vi "LakeShore 340 Controller.vi"(0 "GBPIB Address":refnum<visa-resource-name>, 1 "Reset (I) (0.0)":dbl min=0.0 max=1000.0 step=0.1 format="%.1f", 2 "Rate (D) (0)":dbl min=0.0 max=1000.0 step=1.0, 3 "Manual Output (0.00)":dbl min=0.0 max=100.0 step=0.01 format="%.2f", 4 "Heater Range (0: Off)":u16(ring) items=["Off", "1", "2", "3", "4", "5"], 5 "error out":errorcluster, 6 "Gain (P) (0.0)":dbl min=0.0 max=1000.0 step=0.1 format="%.1f", 7 "Setpoint (0.0)":dbl min=-273.0 max=300000.0 step=0.0001 format="%#.2g", 8 "Loop (0: 1)":u16(ring) items=["1", "2"], 9 "Input (0: A)":u16(ring) items=["A", "B", "C", "D"], 10 "Delay After Config":u32=1000 min=1000 max=99999 step=1) -> (14 "GBPIB Address 2":refnum<visa-resource-name>, 15 "Celsius":dbl min=-273.16 max=1372.0 step=1e-05 format="%#_5g", 16 "K":dbl min=0.0 max=1645.0 step=1e-05 format="%^#_5g", 17 "Ohm":dbl min=-7.5 max=300000.0 step=1e-05 format="%^#_6g", 18 "Heater Output":dbl(slide) min=0.0 max=100.0 step=0.01 scale=0.0..100.0 scale format="%.2f", 19 "error":errorcluster)   [LabVIEW 2019]
doc: "This VI was designed to demonstrate typical usage of sub vi's containing the more common 340 functions.\n\nThis example configures the loop and setpoint of the instrument, allows for a delay, and then reads sensor and heater output data. The user is given the option of just reading data and not configuring the instrument."
uses:
  NHMFL Optics/Globals and TypeDefs/Type Definitions.llb/3 way Status.ctl
  <vilib>/Analysis/baseanly.llb/Mean (DBL).vi
  <vilib>/Analysis/2dsp.llb/Power Spectrum (DBL).vi
  NHMFL Optics/Globals and TypeDefs/gStatus.vi
  NHMFL Optics/Globals and TypeDefs/gTemperature.vi
  <vilib>/Analysis/NI_AALPro.lvlib
  <vilib>/Analysis/NI_AALBase.lvlib
panel:
  out "K plot_t":dbl(graph)
  out "K plot":dbl(graph)
  in  "Tab Control":enum32{"Temperatures", "Configuration", "Misc"}(tab)
  in  "Tolerance":dbl=0.1 min=-273.0 max=300000.0 step=0.0001 format="%#.2g"
  out "Temperature":T1(graph)
  in  "Pause Reading":bool
  in  "AbortChangeTemp":bool
  in  "Reading Rate (ms)":u32=500
  in  "CalibrationTable":bool
  in  "Time-out (s)":dbl
  in  "Manual Advancing":bool
  in  "SetPID":bool
  out "Temperature Control state":T2(ring)
  out "XY Graph":cluster{dbl[], dbl[]}(graph)
  out "Peak time (point)":dbl
  in  "FFT":bool
  in  "stop":bool
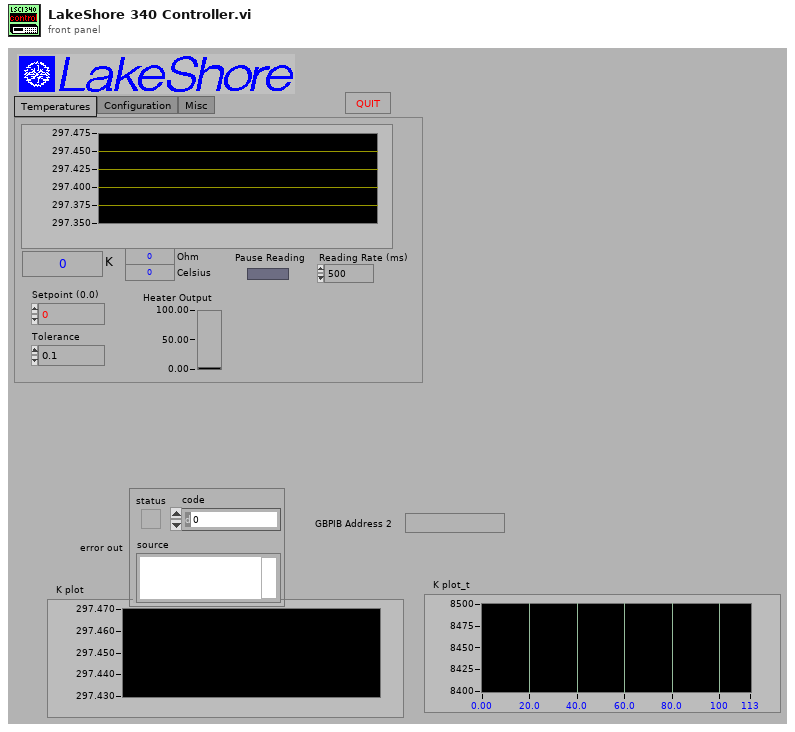
[diagram p1: front panel]
types:
  T1 = cluster{"History Data":dbl[], "History Data":dbl[]}
  T2 = enum16{"--Quit--", "Error", "Init", "Ready", "Set PID", "Set Setpoint", "Curve Manager"}
  T3 = typedef "3 way Status.ctl" = u8
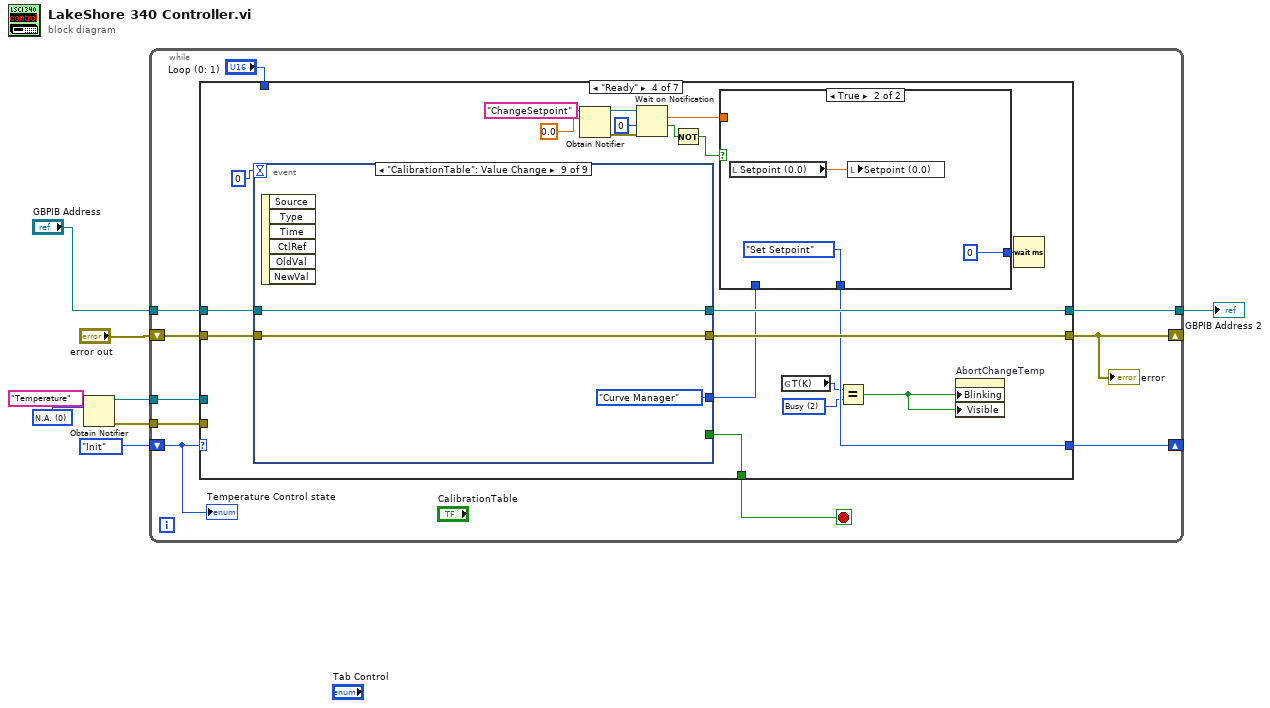
[diagram p0: block diagram]
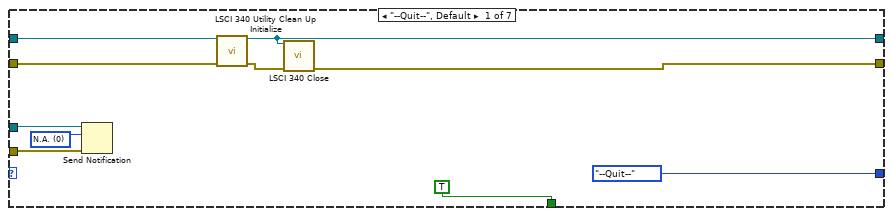
[diagram p2: hidden frame]
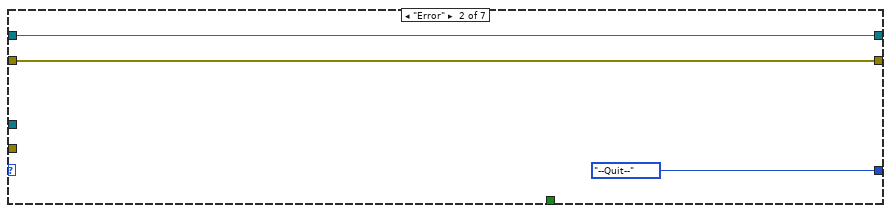
[diagram p3: hidden frame]
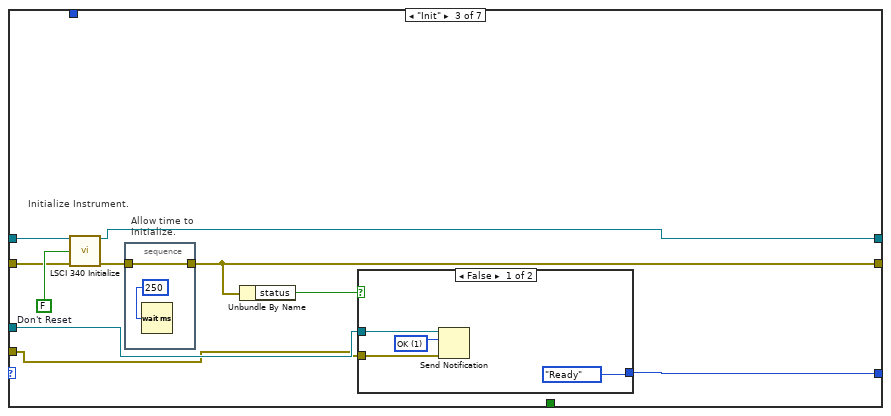
[diagram p4: hidden frame]
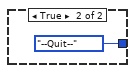
[diagram p5: hidden frame]
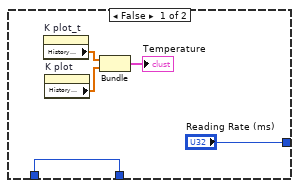
[diagram p6: hidden frame]
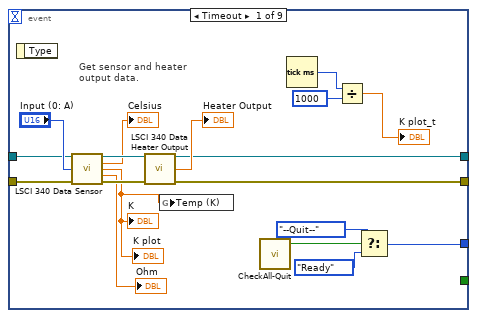
[diagram p7: hidden frame]
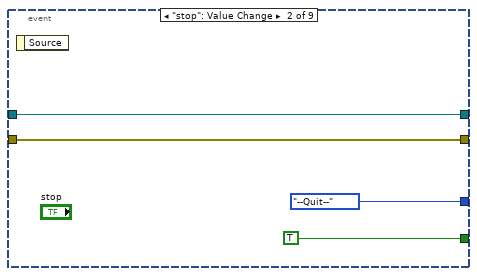
[diagram p8: hidden frame]
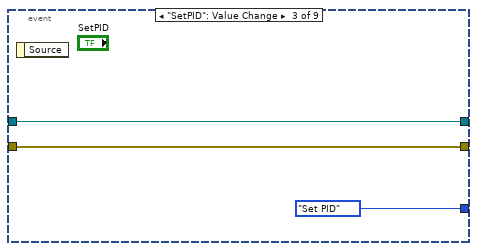
[diagram p9: hidden frame]
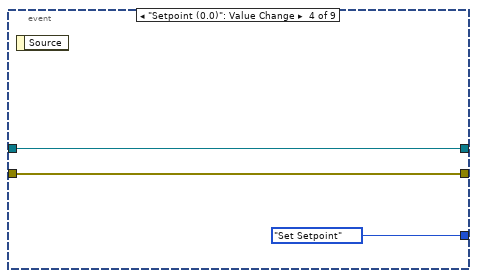
[diagram p10: hidden frame]
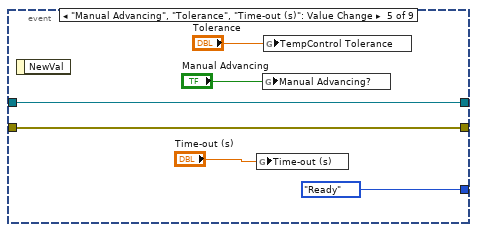
[diagram p11: hidden frame]
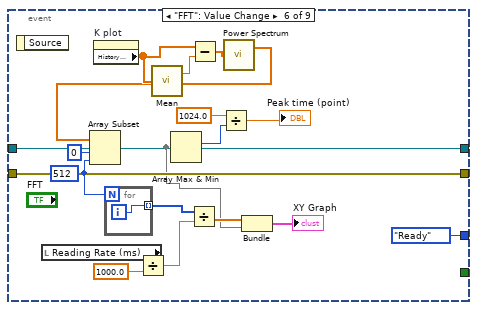
[diagram p12: hidden frame]
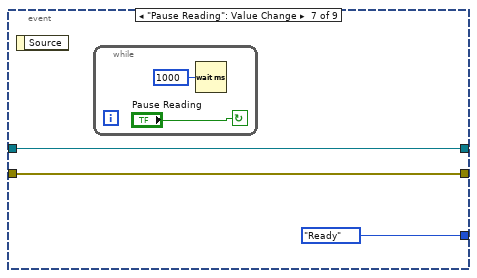
[diagram p13: hidden frame]
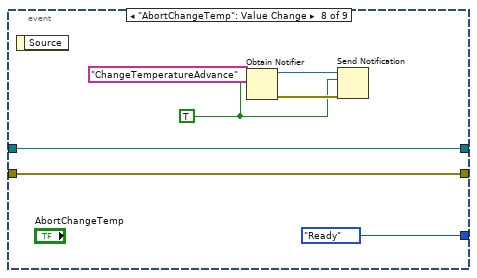
[diagram p14: hidden frame]
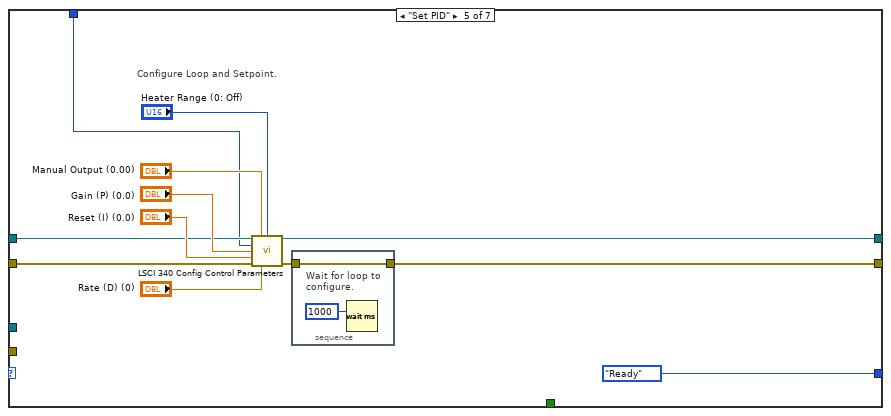
[diagram p15: hidden frame]
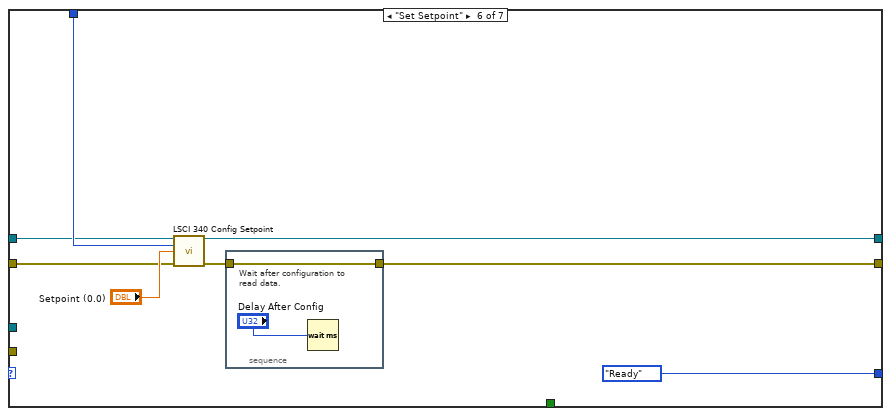
[diagram p16: hidden frame]
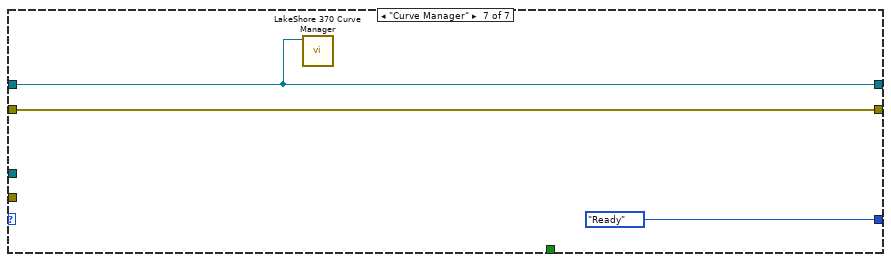
[diagram p17: hidden frame]
diagram:
  w7 = T3 0 items=["N.A.", "OK", "Busy", "Done"] ("Saving")
  n1 = Obtain Notifier(name (unnamed)="Temperature", notification data type=w7) -> (notifier out=w5:refnum<notifier>, error out=w4:errorcluster)  [unwired: 2 in, 1 out]
  n2 = while {
    tunnel: "GBPIB Address" -> [w18]
    shift-right: [w15] -> _
    shift-left: "error out" -> [w17]
    tunnel: [w14] -> w1
    shift-right: [w13] -> _
    shift-left: T2."Init" ("Temperature Control state") -> [w12]
    tunnel: w5 -> [w10]
    tunnel: w4 -> [w9]
    stop <- w11 stop-if-true
    n3 = case shown="\"Ready\"" w12 {
      tunnel: w17 -> [w24 w30 w39 w68 w157 w165 w172]
      tunnel: w18 -> [w25 w31 w33 w67 w153 w163 w170]
      tunnel: [w28 w30 w38 w65 w148 w161 w172] -> w15
      tunnel: [w23 w31 w32 w66 w147 w162 w170] -> w14
      tunnel: "Loop (0: 1)" -> [_ _ _ _ w149 w164 _]
      tunnel: [T2."--Quit--" ("Temperature Control state") T2."--Quit--" ("Temperature Control state") w36 w53 T2."Ready" ("Temperature Control state") T2."Ready" ("Temperature Control state") T2."Ready" ("Temperature Control state")] -> w13
      tunnel: [TRUE ("stop") _ _ w63 _ _ _] -> w11
      tunnel: w10 -> [w20 _ w35 _ _ _ _]
      tunnel: w9 -> [w19 _ w34 _ _ _ _]
      frame "--Quit--", Default {
        w21 = T3 0 items=["N.A.", "OK", "Busy", "Done"] ("notification")
        n4 = Send Notification(notification=w21, notifier=w20, error in (no error)=w19) -> ()  [unwired: 2 out]
        n5 = call "LSCI 340 Utility Clean Up Initialize.vi"("VISA session"=w25, "error in (no error)"=w24) -> ("dup VISA session"=w23:refnum<visa-resource-name>, "error out"=w22:errorcluster)  [unwired: 12 in]
        n6 = call "LSCI 340 Close.vi"("VISA session"=w23, "error in (no error)"=w22) -> ("error out"=w28:errorcluster)  [unwired: 13 in]
      }
      frame "Error" {
      }
      frame "Init" {
        w40 = FALSE  # Don't Reset
        # "Allow time to\nInitialize."
        # "Initialize Instrument."
        n7 = call "LSCI 340 Initialize.vi"("Instr. Descriptor (GPIB::12)"=w33, "Reset (T: Reset)"=w40, "error in (no error)"=w39) -> ("VISA session"=w32:refnum<visa-resource-name>, "error out"=w41:errorcluster)  [unwired: 11 in]
        n8 = stacked-sequence {
          tunnel: w41 -> [w47]
          tunnel: [w47] -> w38
          frame #0 {
            n9 = Wait (ms)(milliseconds to wait=u32 250) -> ()  [unwired: 1 out]
          }
        }
        n10 = Unbundle By Name(w38) -> ("status"=w37:bool)
        n11 = case shown="False" w37 {
          tunnel: [T2."Ready" ("Temperature Control state") T2."--Quit--" ("Temperature Control state")] -> w36
          tunnel: w35 -> [w44 _]
          tunnel: w34 -> [w43 _]
          frame False {
            w42 = T3 1 items=["N.A.", "OK", "Busy", "Done"] ("notification")
            n12 = Send Notification(notification=w42, notifier=w44, error in (no error)=w43) -> ()  [unwired: 2 out]
          }
          frame True {
          }
        }
      }
      frame "Ready" {
        w50 = T3 2 items=["N.A.", "OK", "Busy", "Done"] ("y")
        n13 = event shown="[8] \"CalibrationTable\": Value Change" {
          selector: _ -> [_ _ _ _ _ _ _ _ _]
          dyn-events: _ -> [_ _ _ _ _ _ _ _ _]
          timeout: 0 -> [_ _ _ _ _ _ _ _ _]
          tunnel: w68 -> [w88 w95 w99 w102 w108 w127 w131 w140 w143]
          tunnel: w67 -> [w87 w96 w100 w103 w109 w128 w132 w141 w144]
          tunnel: [w86 w96 w100 w103 w109 w128 w132 w141 w144] -> w66
          tunnel: [w85 w95 w99 w102 w108 w127 w131 w140 w143] -> w65
          tunnel: [_ TRUE ("stop") _ _ _ _ _ _ _] -> w63
          tunnel: [w82 T2."--Quit--" ("Temperature Control state") T2."Set PID" ("Temperature Control state") T2."Set Setpoint" ("Temperature Control state") T2."Ready" ("Temperature Control state") T2."Ready" ("Temperature Control state") T2."Ready" ("Temperature Control state") T2."Ready" ("Temperature Control state") T2."Curve Manager" ("Temperature Control state")] -> w54
          event Timeout {
            # "Get sensor and heater\noutput data."
            n14 = event-data() -> ()  [unwired: 1 in, 1 out]
            n15 = call "LSCI 340 Data Sensor.vi"("VISA session"=w87, "Input (0: A)"="Input (0: A)", "error in (no error)"=w88) -> ("dup VISA session"=w92:refnum<visa-resource-name>, "Celsius Reading"=→"Celsius":dbl, "Kelvin Reading"=w84:dbl, "Sensor Units Reading"=→"Ohm":dbl, "error out"=w93:errorcluster)  [unwired: 8 in]
            "K" <- w84
            "K plot" <- w84
            n16 = call "LSCI 340 Data Heater Output.vi"("VISA session"=w92, "error in (no error)"=w93) -> ("dup VISA session"=w86:refnum<visa-resource-name>, "Heater Output"=→"Heater Output":dbl, "error out"=w85:errorcluster)  [unwired: 11 in]
            n17 = global write "gTemperature.vi" "Temp (K)"(w84) -> ()
            n18 = call "CheckAll-Quit.vi"() -> ("All-Quit"=w83:bool)  [unwired: 3 in]
            n19 = Tick Count (ms)() -> (millisecond timer value=w79:u32)
            n20 = Divide(x=w79, y=u32 1000) -> (x/y=→"K plot_t":dbl)
            n21 = Select(t=T2."--Quit--", s=w83, f=T2."Ready" ("Temperature Control state")) -> (s? t:f=w82:T2)
          }
          event "stop": Value Change {
            n22 = event-data() -> ()  [unwired: 1 in, 1 out]
          }
          event "SetPID": Value Change {
            n23 = event-data() -> ()  [unwired: 1 in, 1 out]
          }
          event "Setpoint (0.0)": Value Change {
            n24 = event-data() -> ()  [unwired: 1 in, 1 out]
          }
          event "Manual Advancing", "Tolerance", "Time-out (s)": Value Change {
            n25 = event-data() -> ()  [unwired: 1 in, 1 out]
            n26 = global write "gTemperature.vi" "Time-out (s)"("Time-out (s)") -> ()
            n27 = global write "gTemperature.vi" "Manual Advancing?"("Manual Advancing") -> ()
            n28 = global write "gTemperature.vi" "TempControl Tolerance"("Tolerance") -> ()
          }
          event "FFT": Value Change {
            w118 = 512 ("length")
            n29 = event-data() -> ()  [unwired: 1 in, 1 out]
            n30 = local read "Reading Rate (ms)"() -> (w116:u32)
            n31 = property on="K plot" class="WFChart (strict)"() -> ("History Data"=w125:dbl[])  [unwired: 2 in, 2 out]
            n32 = for {
              N: w118 -> [_]
              tunnel: [w130] -> w117 mode=indexing
              i -> [w130]
            }
            n33 = Divide(x=w116, y=1000.0) -> (x/y=w112:dbl)
            n34 = call-poly <vilib>:"Mean.vi"("X"=w125) -> ("mean"=w126:dbl)  [unwired: 1 out]
            n35 = Divide(x=w117, y=w112) -> (x/y=w115:dbl[])
            n36 = Subtract(x=w125, y=w126) -> (x-y=w124:dbl[])
            n37 = call-poly <vilib>:"Power Spectrum.vi"("X"=w124) -> ("Power Spectrum"=w120:dbl[])  [unwired: 1 out]
            n38 = Array Subset(array=w120, index=0, length=w118) -> (w114:dbl[])
            n39 = Array Max & Min(array=w114) -> (max index (indices)=w122:i32)  [unwired: 3 out]
            n40 = Divide(x=1024.0, y=w122) -> (x/y=→"Peak time (point)":dbl)
            n41 = Bundle(w115, w114) -> (→"XY Graph":cluster{dbl[], dbl[]})  [unwired: 1 in]
          }
          event "Pause Reading": Value Change {
            n42 = event-data() -> ()  [unwired: 1 in, 1 out]
            n43 = while {
              stop <- "Pause Reading" continue-if-true
              n44 = Wait (ms)(milliseconds to wait=u32 1000) -> ()  [unwired: 1 out]
            }
          }
          event "AbortChangeTemp": Value Change {
            w136 = TRUE ("notification")
            n45 = event-data() -> ()  [unwired: 1 in, 1 out]
            n46 = Obtain Notifier(name (unnamed)="ChangeTemperatureAdvance", notification data type=w136) -> (notifier out=w138:refnum<notifier>, error out=w137:errorcluster)  [unwired: 2 in, 1 out]
            n47 = Send Notification(notification=w136, notifier=w138, error in (no error)=w137) -> ()  [unwired: 2 out]
          }
          event "CalibrationTable": Value Change {
            n48 = event-data() -> ()  [unwired: 1 in, 6 out]
          }
        }
        n49 = Obtain Notifier(name (unnamed)="ChangeSetpoint", notification data type=0.0) -> (notifier out=w58:refnum<notifier>, error out=w57:errorcluster)  [unwired: 2 in, 1 out]
        n50 = Wait on Notification(notifier=w58, timeout in ms (-1)=0, error in (no error)=w57) -> (notification=w55:dbl, timed out?=w59:bool)  [unwired: 1 in, 2 out]
        n51 = Not(x=w59) -> (.not. x?=w56:bool)
        n52 = case shown="True" w56 {
          tunnel: w55 -> [_ _]
          tunnel: w54 -> [w73 _]
          tunnel: [w73 T2."Set Setpoint" ("Temperature Control state")] -> w53
          tunnel: ["Reading Rate (ms)" u32 0 ("Refresh (ms)")] -> w52
          frame False {
            n53 = property on="K plot_t" class="WFChart (strict)"() -> ("History Data"=w72:dbl[])  [unwired: 2 in, 2 out]
            n54 = property on="K plot" class="WFChart (strict)"() -> ("History Data"=w71:dbl[])  [unwired: 2 in, 2 out]
            n55 = Bundle("History Data"=w72, "History Data"=w71) -> (→"Temperature":T1)  [unwired: 1 in]
          }
          frame True {
            n56 = local read "Setpoint (0.0)"() -> (w74:dbl)
            n57 = local write "Setpoint (0.0)"(w74) -> ()
          }
        }
        n58 = global read "gStatus.vi" "T(K)"() -> (w51:T3)
        n59 = Equal?(x=w51, y=w50) -> (x = y?=w49:bool)
        n60 = property on="AbortChangeTemp" class="Bool"("Blinking"=w49, "Visible"=w49) -> ()  [unwired: 2 in, 2 out]
        n61 = Wait (ms)(milliseconds to wait=w52) -> ()  [unwired: 1 out]
      }
      frame "Set PID" {
        # "Configure Loop and Setpoint."
        n62 = call "LSCI 340 Config Control Parameters.vi"("VISA session"=w153, "Manual Output (0.00)"="Manual Output (0.00)", "Heater Range (0: Off)"="Heater Range (0: Off)", "Loop (0: 1)"=w149, "Gain (P) (0.0)"="Gain (P) (0.0)", "Reset (I) (0.0)"="Reset (I) (0.0)", "error in (no error)"=w157, "Rate (D) (0)"="Rate (D) (0)") -> ("dup VISA session"=w147:refnum<visa-resource-name>, "error out"=w150:errorcluster)  [unwired: 6 in]
        n63 = stacked-sequence {
          tunnel: w150 -> [w158]
          tunnel: [w158] -> w148
          frame #0 {
            # "Wait for loop to \nconfigure."
            n64 = Wait (ms)(milliseconds to wait=u32 1000) -> ()  [unwired: 1 out]
          }
        }
      }
      frame "Set Setpoint" {
        n65 = call "LSCI 340 Config Setpoint.vi"("VISA session"=w163, "Loop (0: 1)"=w164, "Setpoint (0.0)"="Setpoint (0.0)", "error in (no error)"=w165) -> ("dup VISA session"=w162:refnum<visa-resource-name>, "error out"=w166:errorcluster)  [unwired: 10 in]
        n66 = stacked-sequence {
          tunnel: w166 -> [w169]
          tunnel: [w169] -> w161
          frame #0 {
            # "Wait after configuration to\nread data."
            n67 = Wait (ms)(milliseconds to wait="Delay After Config") -> ()  [unwired: 1 out]
          }
        }
      }
      frame "Curve Manager" {
        n68 = call "LakeShore 370 Curve Manager.vi"("VISA session"=w170) -> ()  [unwired: 11 in]
      }
    }
    "error" <- w15
    "Temperature Control state" <- w12
  }
  "GBPIB Address 2" <- w1
